vi "To Pretty String (Array).vi"(6 "pretty print? (T)":bool=TRUE, 7 "enable LabVIEW extensions? (T)":bool=TRUE, 8 "error in (no error)":errorcluster, 11 "JSON Value in":refnum<class "JSON Value.lvclass">) -> (0 "error out":errorcluster, 3 "Pretty Print String":string)   [LabVIEW 2016, in "JSON Value.lvclass"]
doc: "Pretty prints the given JSON data in an easier to read format."
uses:
  JSON Value.lvclass
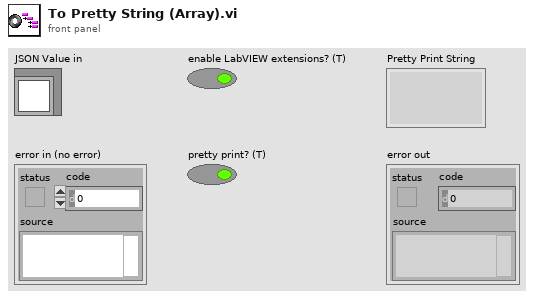
[diagram p1: front panel]
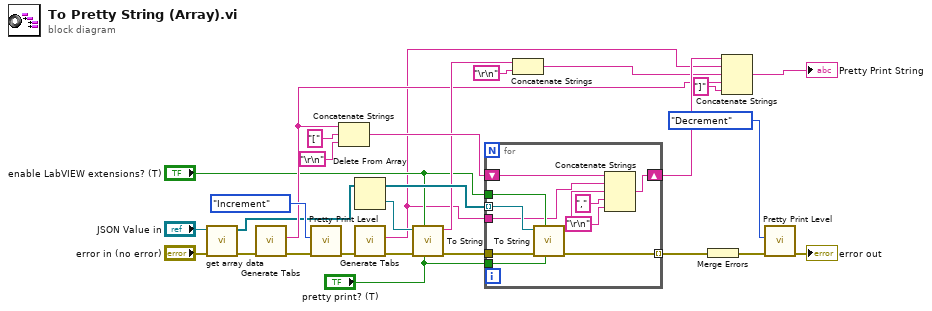
[diagram p0: block diagram]
diagram:
  n1 = call "get array data.vi"("error in (no error)"="error in (no error)", "JSON Value in"="JSON Value in") -> ("error out"=w3:errorcluster, "JSON Array out"=w7:refnum<class "JSON Value.lvclass">[])  [unwired: 8 in]
  n2 = call "Generate Tabs.vi"("error in (no error)"=w3) -> ("error out"=w24:errorcluster, "Tabs"=w10:string)  [unwired: 9 in]
  n3 = call "Pretty Print Level.vi"("error in (no error)"=w24, "Action"=enum16{"Increment", "Decrement", "Get", "Reset"}."Increment") -> ("error out"=w19:errorcluster)  [unwired: 8 in, 1 out]
  n4 = Concatenate Strings(w10, "[" ("string"), "\r\n") -> (w25:string)
  n5 = Delete From Array(array=w7) -> (deleted portion=w17:refnum<class "JSON Value.lvclass">, array with subset deleted=w18:refnum<class "JSON Value.lvclass">[])  [unwired: 2 in]
  n6 = call "Generate Tabs.vi"("error in (no error)"=w19) -> ("error out"=w9:errorcluster, "Tabs"=w1:string)  [unwired: 9 in]
  n7 = call "To String.vi"("pretty print? (T)"="pretty print? (T)", "enable LabVIEW extensions? (T)"="enable LabVIEW extensions? (T)", "error in (no error)"=w9, "JSON Value in"=w17) -> ("error out"=w8:errorcluster, "String"=w16:string)  [unwired: 6 in]
  n8 = for {
    tunnel: w18 -> [w39] mode=indexing
    tunnel: w8 -> [w38]
    tunnel: [w37] -> w28 mode=indexing
    shift-right: [w33] -> w14
    shift-left: w25 -> [w32]
    tunnel: w1 -> [w29]
    tunnel: "enable LabVIEW extensions? (T)" -> [w31]
    tunnel: "pretty print? (T)" -> [w30]
    n9 = call "To String.vi"("pretty print? (T)"=w30, "enable LabVIEW extensions? (T)"=w31, "error in (no error)"=w38, "JSON Value in"=w39) -> ("error out"=w37:errorcluster, "String"=w36:string)  [unwired: 6 in]
    n10 = Concatenate Strings(w32, w29, w36, "," ("string"), "\r\n") -> (w33:string)
  }
  n11 = Concatenate Strings(w16, "\r\n") -> (w13:string)
  n12 = Merge Errors(w28) -> (w23:errorcluster)
  n13 = Concatenate Strings(w14, w1, w13, w10, "]" ("string")) -> (→"Pretty Print String":string)
  n14 = call "Pretty Print Level.vi"("error in (no error)"=w23, "Action"=enum16{"Increment", "Decrement", "Get", "Reset"}."Decrement") -> ("error out"=→"error out":errorcluster)  [unwired: 8 in, 1 out]
